vi "TelemetryServer_QueueStop.vi"(3 "Telemetry queues":refnum<queue>[](array[refnum]), 7 "Queue references":refnum<vi>[](array[refnum]), 9 "Error out":errorcluster caption="Error in (no error)") -> (6 "error out":errorcluster)   [LabVIEW 2009]
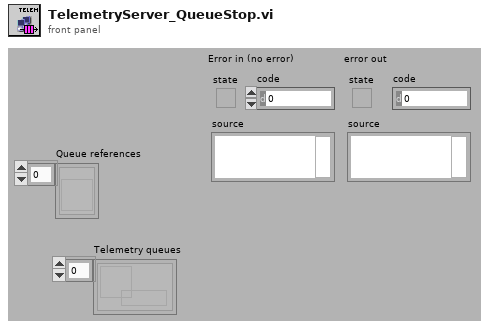
[diagram p1: front panel]
types:
  T1 = enum32{"Bad", "Idle", "Run top level", "Running"}
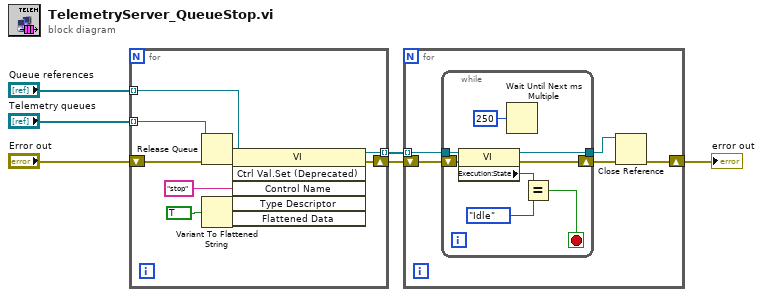
[diagram p0: block diagram]
diagram:
  n1 = for {
    tunnel: [w16] -> w6 mode=indexing
    tunnel: "Telemetry queues" -> [w8] mode=indexing
    tunnel: "Queue references" -> [w7] mode=indexing
    shift-right: [w15] -> w5
    shift-left: "Error out" -> [w9]
    n2 = Release Queue(queue=w8, error in (no error)=w9) -> (error out=w10:errorcluster)  [unwired: 3 out]
    n3 = Variant To Flattened String(Variant=TRUE) -> (data string=w13:string, 1:w12:i16[])
    n4 = invoke class="VI" method="Ctrl Val.Set (Deprecated)"(reference=w7, error in=w10, "Control Name"="stop" ("Nom de la commande"), "Type Descriptor"=w12, "Flattened Data"=w13) -> (reference out=w16:refnum<vi>, error out=w15:errorcluster)  [unwired: 1 in, 4 out]
  }
  n5 = for {
    tunnel: w6 -> [w19] mode=indexing
    shift-right: [w17] -> w3
    shift-left: w5 -> [w18]
    n6 = while {
      tunnel: w19 -> [w28]
      tunnel: [w23] -> w21
      shift-right: [w22] -> w20
      shift-left: w18 -> [w29]
      stop <- w24 stop-if-true
      n7 = property class="VI"(reference=w28, error in=w29) -> (reference out=w23:refnum<vi>, error out=w22:errorcluster, "Execution:State"=w27:T1)
      n8 = Wait Until Next ms Multiple(millisecond multiple=u32 250 ("n millisecondes")) -> ()  [unwired: 1 out]
      n9 = Equal?(x=w27, y=T1."Idle" ("Exécution : état")) -> (x = y?=w24:bool)
    }
    n10 = Close Reference(reference=w21, error in (no error)=w20) -> (error out=w17:errorcluster)
  }
  "error out" <- w3
